vi "Steppers_and_Scanners_control_6_15.vi"(1 "ANC300 address":refnum<visa-resource-name>="COM8") -> (18 "Serial":string="ANC300B-C-2133-4009033")   [LabVIEW 2024]
panel:
  in  "wait time (ms)":u32=300
  out "2: Voltage Reading":dbl format="%#_13g"
  out "1: Voltage Reading":dbl format="%#_13g"
  in  "Set/Read":bool=TRUE
  in  "Stepper 4":bool
  in  "4: number of steps":i32=1
  in  "4: stepping direction":bool=TRUE
  in  "4: AC Voltage":dbl=60.0 min=0.0 format="%.1f"
  in  "4: AC frequency":dbl=300.0 min=0.0 format="%.1f"
  in  "Stepper 3":bool
  in  "3: number of steps":i32=1
  in  "3: stepping direction":bool=TRUE
  in  "3: AC Voltage":dbl=60.0 min=0.0 format="%.1f"
  in  "3: AC frequency":dbl=300.0 min=0.0 format="%.1f"
  in  "2: ms to wait":u32=30
  in  "2: Offset Voltage":dbl min=0.0 max=150.0 format="%.2g"
  in  "1: ms to wait":u32=30
  in  "1: Offset Voltage":dbl min=0.0 max=150.0 format="%.2f"
  # "scanner limits: 150V at 2K. 60V at 300K"
  # "Scanner 1"
  # "Scanner 2"
  # "59"
  # "66"
  # "22, 18"
  # "1. Shouldn't have to change the ms to wait times. \n2. If the piezos aren't moving, it's probably because they need to be exercised first. Best to do that manually\nwith the switches on the board or by moving it here several steps at a time with a high AC voltage. If it doesn't move, you have to rerun the file because it is waiting for it to move and will get stuck there if it isn't moving.\n3. Set 'low temperature' or 'high temperature' limits on the controller manually. You can't do that remotely.  DONT GO ABOVE 60V"
  # "Move Stepper 3 Once"
  # "Move Stepper 4 Once"
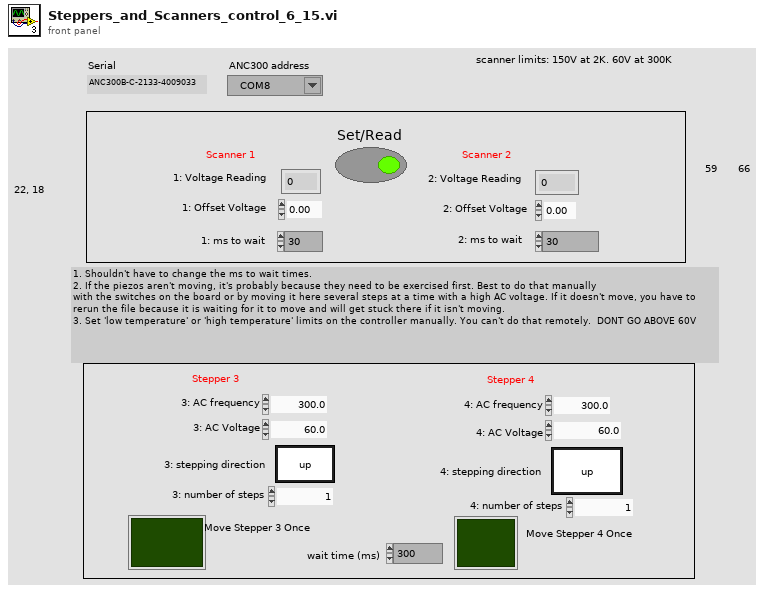
[diagram p1: front panel]
types:
  T1 = cluster{"error ":bool, "error number":i32, "error code":string}
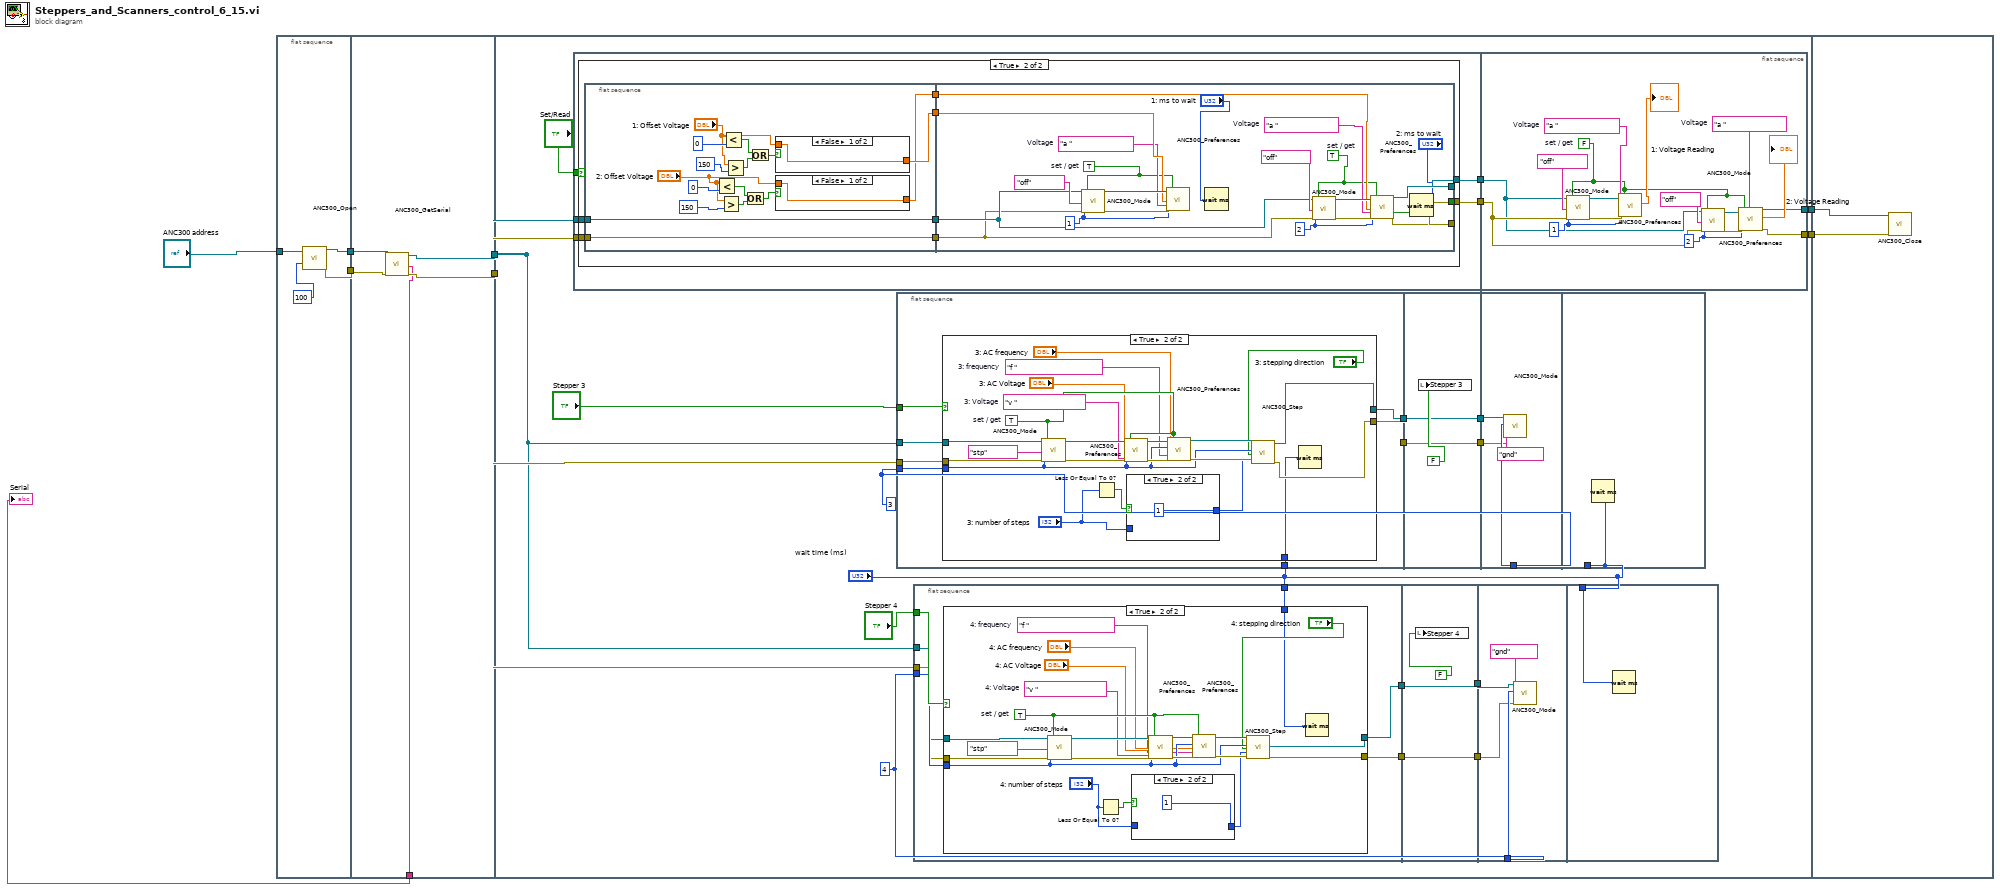
[diagram p0: block diagram]
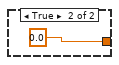
[diagram p3: hidden frame]
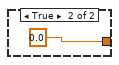
[diagram p4: hidden frame]
diagram:
  n1 = flat-sequence {
    tunnel: "ANC300 address" -> [w11]
    tunnel: [w12] -> w8
    tunnel: [w10] -> w7
    tunnel: w8 -> [w17]
    tunnel: w7 -> [w16]
    tunnel: [w15] -> w6
    tunnel: [w14] -> w5
    tunnel: [w13] -> w4
    tunnel: w6 -> [w34]
    tunnel: w5 -> [w35]
    tunnel: [w19] -> w2
    tunnel: [w18] -> w1
    tunnel: w2 -> [w194]
    tunnel: w1 -> [w193]
    frame #0 {
      n2 = call "ANC300_Open.vi"("ANC300 Communication Port In"=w11, "milliseconds to wait"=u32 100 ("millisecond timer value")) -> ("ANC300 Communication Port Out"=w12:refnum<visa-resource-name>, "error out"=w10:T1)  [unwired: 13 in, 3 out]
    }
    frame #1 {
      n3 = call "ANC300_GetSerial.vi"("ANC300 Communication Port In"=w17, "error in"=w16) -> ("ANC300 Communication Port Out"=w15:refnum<visa-resource-name>, "Serial"=w13:string, "error out"=w14:T1)  [unwired: 10 in, 5 out]
    }
    frame #2 {
      w33 = 3
      w36 = 4
      n4 = flat-sequence {
        tunnel: w35 -> [w42]
        tunnel: w34 -> [w41]
        tunnel: "Set/Read" -> [w40]
        tunnel: [w39] -> w26
        tunnel: [w38] -> w25
        tunnel: w26 -> [w99]
        tunnel: w25 -> [w100]
        tunnel: [w95] -> w19
        tunnel: [w94] -> w18
        frame #0 {
          n5 = case shown="True" w40 {
            tunnel: w42 -> [w43 w52]
            tunnel: w41 -> [w44 w47]
            tunnel: [w44 w49] -> w39
            tunnel: [w43 w48] -> w38
            frame False {
            }
            frame True {
              n6 = flat-sequence {
                tunnel: w52 -> [w67]
                tunnel: w47 -> [w68]
                tunnel: [w68] -> w51
                tunnel: [w67] -> w50
                tunnel: [w60] -> w46
                tunnel: [w54] -> w45
                tunnel: w51 -> [w77]
                tunnel: w50 -> [w76]
                tunnel: [w75] -> w49
                tunnel: [w74] -> _
                tunnel: [w73] -> w48
                tunnel: w46 -> [w91]
                tunnel: w45 -> [w84]
                frame #0 {
                  n7 = Less?(x="2: Offset Voltage", y=0) -> (x < y?=w56:bool)
                  n8 = Greater?(x="2: Offset Voltage", y=150) -> (0:w57:bool)
                  n9 = Less?(x="1: Offset Voltage", y=0) -> (x < y?=w64:bool)
                  n10 = Greater?(x="1: Offset Voltage", y=150) -> (0:w63:bool)
                  n11 = Or(x=w56, y=w57) -> (x .or. y?=w55:bool)
                  n12 = Or(x=w64, y=w63) -> (x .or. y?=w62:bool)
                  n13 = case shown="False" w62 {
                    tunnel: "1: Offset Voltage" -> [w71 _]
                    tunnel: [w71 0.0] -> w60
                    frame False {
                    }
                    frame True {
                    }
                  }
                  n14 = case shown="False" w55 {
                    tunnel: "2: Offset Voltage" -> [w69 _]
                    tunnel: [w69 0.0] -> w54
                    frame False {
                    }
                    frame True {
                    }
                  }
                }
                frame #1 {
                  w78 = 2
                  w79 = 1
                  w80 = TRUE  # set / get
                  w83 = "a "  # Voltage
                  w87 = TRUE  # set / get
                  w90 = "a "  # Voltage
                  n15 = call "ANC300_Mode.vi"("ANC300 Communication Port In"=w77, "Axis"=w79, "axis mode in"="off", "error in"=w76, "set / get"=w87) -> ("ANC300 Communication Port Out"=w93:refnum<visa-resource-name>, "error out"=w92:T1)  [unwired: 8 in, 5 out]
                  n16 = call "ANC300_Preferences.vi"("ANC300 Communication Port In"=w93, "Axis"=w79, "value in"=w91, "parameter"=w90, "error in"=w92, "set / get"=w87) -> ()  [unwired: 6 in, 8 out]
                  n17 = Wait (ms)(milliseconds to wait="1: ms to wait") -> ()  [unwired: 1 out]
                  n18 = call "ANC300_Mode.vi"("ANC300 Communication Port In"=w77, "Axis"=w78, "axis mode in"="off", "error in"=w76, "set / get"=w80) -> ("ANC300 Communication Port Out"=w86:refnum<visa-resource-name>, "error out"=w85:T1)  [unwired: 8 in, 5 out]
                  n19 = call "ANC300_Preferences.vi"("ANC300 Communication Port In"=w86, "Axis"=w78, "value in"=w84, "parameter"=w83, "error in"=w85, "set / get"=w80) -> ("ANC300 Communication Port Out"=w75:refnum<visa-resource-name>, "transfer ok"=w74:bool, "error out"=w73:T1)  [unwired: 6 in, 5 out]
                  n20 = Wait (ms)(milliseconds to wait="2: ms to wait") -> ()  [unwired: 1 out]
                }
              }
            }
          }
        }
        frame #1 {
          w101 = 2
          w102 = 1
          w104 = "a "  # Voltage
          w96 = FALSE  # set / get
          w108 = "a "  # Voltage
          n21 = call "ANC300_Mode.vi"("ANC300 Communication Port In"=w99, "Axis"=w102, "axis mode in"="off", "error in"=w100, "set / get"=w96) -> ("ANC300 Communication Port Out"=w110:refnum<visa-resource-name>, "error out"=w109:T1)  [unwired: 8 in, 5 out]
          n22 = call "ANC300_Preferences.vi"("ANC300 Communication Port In"=w110, "Axis"=w102, "parameter"=w108, "error in"=w109, "set / get"=w96) -> ("value out"=→"1: Voltage Reading":dbl)  [unwired: 7 in, 7 out]
          n23 = call "ANC300_Mode.vi"("ANC300 Communication Port In"=w99, "Axis"=w101, "axis mode in"="off", "error in"=w100, "set / get"=w96) -> ("ANC300 Communication Port Out"=w106:refnum<visa-resource-name>, "error out"=w105:T1)  [unwired: 8 in, 5 out]
          n24 = call "ANC300_Preferences.vi"("ANC300 Communication Port In"=w106, "Axis"=w101, "parameter"=w104, "error in"=w105, "set / get"=w96) -> ("ANC300 Communication Port Out"=w95:refnum<visa-resource-name>, "value out"=→"2: Voltage Reading":dbl, "error out"=w94:T1)  [unwired: 7 in, 5 out]
        }
      }
      n25 = flat-sequence {
        tunnel: "Stepper 3" -> [w117]
        tunnel: w33 -> [w116]
        tunnel: w34 -> [w115]
        tunnel: w35 -> [w114]
        tunnel: [w113] -> w28
        tunnel: [w112] -> w23
        tunnel: "wait time (ms)" -> [w111]
        tunnel: [w145] -> w29
        tunnel: w28 -> [w145]
        tunnel: [w144] -> w24
        tunnel: w23 -> [w144]
        tunnel: w33 -> [w149]
        tunnel: w29 -> [w148]
        tunnel: w24 -> [w147]
        tunnel: "wait time (ms)" -> [w151]
        tunnel: [w151] -> _
        frame #0 {
          n26 = case shown="True" w117 {
            tunnel: w115 -> [w119 w141]
            tunnel: w116 -> [_ w133]
            tunnel: w114 -> [w118 w138]
            tunnel: [w119 w132] -> w113
            tunnel: [w118 w124] -> w112
            tunnel: w111 -> [_ w123]
            frame False {
            }
            frame True {
              w126 = "v "  # 3: Voltage
              w128 = "f "  # 3: frequency
              w131 = TRUE  # set / get
              n27 = call "ANC300_Mode.vi"("ANC300 Communication Port In"=w141, "Axis"=w133, "axis mode in"="stp", "error in"=w138, "set / get"=w131) -> ("ANC300 Communication Port Out"=w140:refnum<visa-resource-name>, "error out"=w137:T1)  [unwired: 8 in, 5 out]
              n28 = Less Or Equal To 0?(x="3: number of steps") -> (x <= 0?=w121:bool)
              n29 = call "ANC300_Preferences.vi"("ANC300 Communication Port In"=w140, "Axis"=w133, "value in"="3: AC Voltage", "parameter"=w126, "error in"=w137, "set / get"=w131) -> ("ANC300 Communication Port Out"=w135:refnum<visa-resource-name>, "error out"=w134:T1)  [unwired: 6 in, 6 out]
              n30 = case shown="True" w121 {
                tunnel: "3: number of steps" -> [w142 _]
                tunnel: [w142 1] -> w120
                frame False {
                }
                frame True {
                }
              }
              n31 = call "ANC300_Preferences.vi"("ANC300 Communication Port In"=w135, "Axis"=w133, "value in"="3: AC frequency", "parameter"=w128, "error in"=w134, "set / get"=w131) -> ("ANC300 Communication Port Out"=w139:refnum<visa-resource-name>, "error out"=w136:T1)  [unwired: 6 in, 6 out]
              n32 = call "ANC300_Step.vi"("ANC300 Communication Port In"=w139, "Axis"=w133, "stepping direction"="3: stepping direction", "number of steps [0=cont.]"=w120, "error in"=w136) -> ("ANC300 Communication Port Out"=w132:refnum<visa-resource-name>, "error out"=w124:T1)  [unwired: 9 in, 4 out]
              n33 = Wait (ms)(milliseconds to wait=w123) -> ()  [unwired: 1 out]
            }
          }
        }
        frame #1 {
          n34 = local write "Stepper 3"(FALSE) -> ()
        }
        frame #2 {
          n35 = call "ANC300_Mode.vi"("ANC300 Communication Port In"=w148, "Axis"=w149, "axis mode in"="gnd" ("3 Stepper x"), "error in"=w147) -> ()  [unwired: 9 in, 7 out]
        }
        frame #3 {
          n36 = Wait (ms)(milliseconds to wait=w151) -> ()  [unwired: 1 out]
        }
      }
      n37 = flat-sequence {
        tunnel: "Stepper 4" -> [w158]
        tunnel: w36 -> [w157]
        tunnel: w34 -> [w156]
        tunnel: w35 -> [w155]
        tunnel: [w154] -> w30
        tunnel: [w153] -> w21
        tunnel: "wait time (ms)" -> [w152]
        tunnel: [w186] -> w31
        tunnel: w30 -> [w186]
        tunnel: [w185] -> w22
        tunnel: w21 -> [w185]
        tunnel: w36 -> [w190]
        tunnel: w31 -> [w189]
        tunnel: w22 -> [w188]
        tunnel: "wait time (ms)" -> [w192]
        frame #0 {
          n38 = case shown="True" w158 {
            tunnel: w156 -> [w160 w182]
            tunnel: w157 -> [_ w174]
            tunnel: w155 -> [w159 w179]
            tunnel: [w160 w173] -> w154
            tunnel: [w159 w165] -> w153
            tunnel: w152 -> [_ w164]
            frame False {
            }
            frame True {
              w170 = "v "  # 4: Voltage
              w168 = "f "  # 4: frequency
              w172 = TRUE  # set / get
              n39 = call "ANC300_Mode.vi"("ANC300 Communication Port In"=w182, "Axis"=w174, "axis mode in"="stp", "error in"=w179, "set / get"=w172) -> ("ANC300 Communication Port Out"=w181:refnum<visa-resource-name>, "error out"=w178:T1)  [unwired: 8 in, 5 out]
              n40 = Less Or Equal To 0?(x="4: number of steps") -> (x <= 0?=w161:bool)
              n41 = case shown="True" w161 {
                tunnel: "4: number of steps" -> [w183 _]
                tunnel: [w183 1] -> w162
                frame False {
                }
                frame True {
                }
              }
              n42 = call "ANC300_Preferences.vi"("ANC300 Communication Port In"=w181, "Axis"=w174, "value in"="4: AC Voltage", "parameter"=w170, "error in"=w178, "set / get"=w172) -> ("ANC300 Communication Port Out"=w176:refnum<visa-resource-name>, "error out"=w175:T1)  [unwired: 6 in, 6 out]
              n43 = call "ANC300_Preferences.vi"("ANC300 Communication Port In"=w176, "Axis"=w174, "value in"="4: AC frequency", "parameter"=w168, "error in"=w175, "set / get"=w172) -> ("ANC300 Communication Port Out"=w180:refnum<visa-resource-name>, "error out"=w177:T1)  [unwired: 6 in, 6 out]
              n44 = call "ANC300_Step.vi"("ANC300 Communication Port In"=w180, "Axis"=w174, "stepping direction"="4: stepping direction", "number of steps [0=cont.]"=w162, "error in"=w177) -> ("ANC300 Communication Port Out"=w173:refnum<visa-resource-name>, "error out"=w165:T1)  [unwired: 9 in, 4 out]
              n45 = Wait (ms)(milliseconds to wait=w164) -> ()  [unwired: 1 out]
            }
          }
        }
        frame #1 {
          n46 = local write "Stepper 4"(FALSE) -> ()
        }
        frame #2 {
          n47 = call "ANC300_Mode.vi"("ANC300 Communication Port In"=w189, "Axis"=w190, "axis mode in"="gnd" ("3 Stepper x"), "error in"=w188) -> ()  [unwired: 9 in, 7 out]
        }
        frame #3 {
          n48 = Wait (ms)(milliseconds to wait=w192) -> ()  [unwired: 1 out]
        }
      }
    }
    frame #3 {
      n49 = call "ANC300_Close.vi"("ANC300 Communication Port In"=w194, "error in"=w193) -> ()  [unwired: 17 in, 1 out]
    }
  }
  "Serial" <- w4
